vi "Создание каждый раз нового файла.vi"   [LabVIEW 2021]
types:
  T1 = enum16{"open", "replace", "create", "open or create", "replace or create", "replace or create with confirmation"}
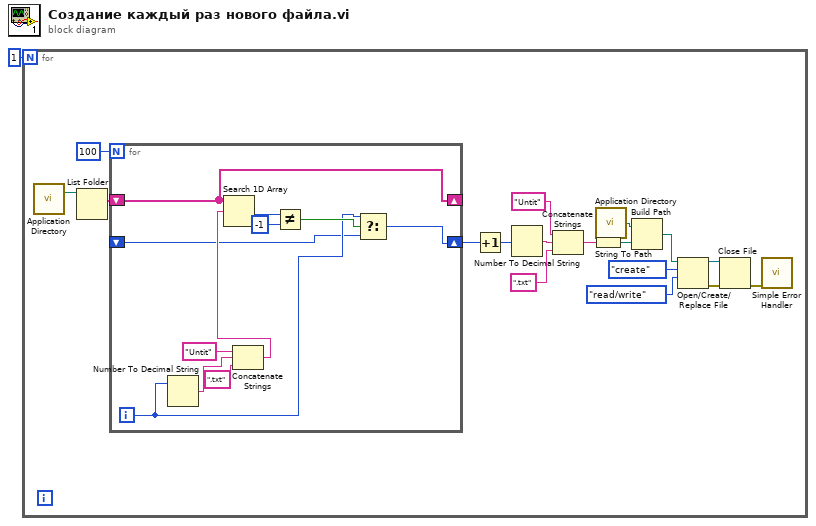
[diagram p0: block diagram]
diagram:
  n1 = for {
    N: 1 -> [_]
    n2 = call <vilib>:"Application Directory.vi"() -> ("Application Directory"=w7:path)
    n3 = List Folder(path=w7) -> (filenames=w6:string[])  [unwired: 3 in, 3 out]
    n4 = for {
      N: 100 -> [_]
      shift-right: [w23] -> _
      shift-left: w6 -> [w23]
      shift-right: [w19] -> w4
      shift-left: _ -> [w20]
      i -> [w21]
      n5 = Number To Decimal String(number=w21) -> (decimal integer string=w27:string)  [unwired: 1 in]
      n6 = Concatenate Strings("Untit" ("string"), w27, ".txt" ("string")) -> (w26:string)
      n7 = Search 1D Array(1D array=w23, element=w26) -> (index of element=w25:i32)  [unwired: 1 in]
      n8 = Not Equal?(x=w25, y=-1) -> (x != y?=w22:bool)
      n9 = Select(t=w21, s=w22, f=w20) -> (s? t:f=w19:i32)
    }
    n10 = Increment(x=w4) -> (x+1=w3:i32)
    n11 = Number To Decimal String(number=w3) -> (decimal integer string=w2:string)  [unwired: 1 in]
    n12 = Concatenate Strings("Untit" ("string"), w2, ".txt" ("string")) -> (w12:string)
    n13 = String To Path(string=w12) -> (path=w13:path)
    n14 = call <vilib>:"Application Directory.vi"() -> ("Application Directory"=w14:path)
    n15 = Build Path(base path=w14, name or relative path=w13) -> (appended path=w15:path)
    n16 = Open/Create/Replace File(file path (use dialog)=w15, operation (0:open)=T1."create", access (0:read/write)=enum16{"read/write", "read-only", "write-only"}."read/write") -> (refnum out=w10:refnum<file>, error out=w9:errorcluster)  [unwired: 3 in, 1 out]
    n17 = Close File(refnum=w10, error in=w9) -> (error out=w16:errorcluster)  [unwired: 1 out]
    n18 = call <vilib>:"Simple Error Handler.vi"("error in (no error)"=w16) -> ()  [unwired: 4 in, 5 out]
  }
